vi "Cheak_time.vi"() -> ()   [LabVIEW 2019]
uses:
  <vilib>/Platform/TimedLoop/XDataNode/timing_clust.ctl
  <vilib>/Platform/TimedLoop/XDataNode/nitl_modes.ctl
  <vilib>/Platform/TimedLoop/XDataNode/wakeup.ctl
  <vilib>/FPGAPlugInAG/cRIO-9040/niLvFpga_Open_cRIO-9040.vi
  <vilib>/rvi/interface/common/dynamic/niFpgaDynamicAddResources.vi
  <vilib>/FPGAPlugInAG/Dynamic/niLvFpga_Reset_Dynamic.vi
  <vilib>/FPGAPlugInAG/Dynamic/niLvFpga_Run_Dynamic.vi
  <vilib>/Utility/error.llb/Error Cluster From Error Code.vi
  <vilib>/rvi/errors/niLvFpgaAdjustHostInterfaceError.vi
  <vilib>/FPGAPlugInAG/Dynamic/niLvFpga_Abort_Dynamic.vi
  <vilib>/FPGAPlugInAG/Dynamic/niLvFpga_Close_Dynamic.vi
  <vilib>/rvi/interface/nirviOpenFPGA/nirviOpenFPGA.xnode
  FPGA Bitfiles/hipabvelocitypro_FPGATarget_FPGADATA_ajS4pduxPJ4.lvbitx
  FPGA/FPGA_DATA.vi
  <vilib>/rvi/interface/nirviMethod/nirviMethod.xnode
  <vilib>/Platform/TimedLoop/XDataNode/XDataNode.xnode
  <vilib>/rvi/interface/nirviReadWriteControl/nirviReadWriteControl.xnode
  <vilib>/rvi/interface/nirviCloseFPGA/nirviCloseFPGA.xnode
  <vilib>/Platform/TimedLoop/XDataNode/XDNodeRunTimeDep.lvlib
  NiFpgaLv.dll
  <vilib>/rvi/interface/Simulation/niFpgaSimulationCallBeginRW.vi
panel:
  out "클러스터":T1
  in  "R_velocity":u32
  in  "Temporal parameters_Negative_L":T2={"Onset start"=0.0, "Onset end"=2.0, "Peak start"=10.0, "Release start"=36.0, "slang"=45.0, "Peak end"=34.0}
  in  "L_velocity":u32
  out "Mod1/CAN0":T3={"timestamp high"=0, "timestamp low"=0, "identifier"=0, "type"=enum."Data Frame", "info A"=0, "info B"=0, "data length"=0, "data"=[0, 0, 0, 0, 0, 0, 0, 0]}
  in  "SAVE":bool
  out "웨이브폼 차트 3":T4(graph)
  in  "정지":bool
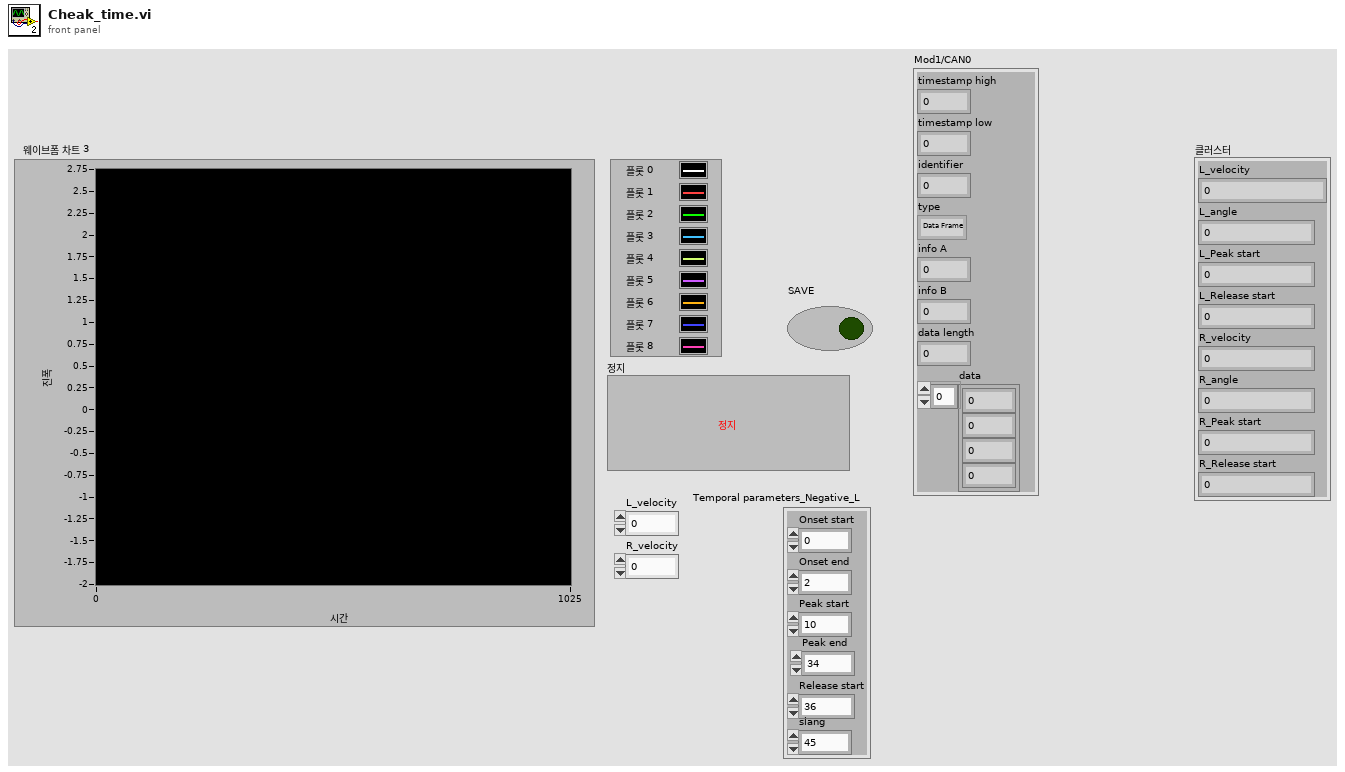
[diagram p1: front panel]
types:
  T1 = cluster{"L_velocity":u32, "L_angle":sgl, "L_Peak start":sgl, "L_Release start":sgl, "R_velocity":u32, "R_angle":sgl, "R_Peak start":sgl, "R_Release start":sgl}
  T2 = cluster{"Onset start":sgl, "Onset end":sgl, "Peak start":sgl, "Release start":sgl, "slang":sgl, "Peak end":sgl}
  T3 = cluster{"timestamp high":u32, "timestamp low":u32, "identifier":u32, "type":enum8{"Data Frame", "Remote Frame", "(reserved)", "(reserved) ", "(reserved)  ", "(reserved)   ", "Bus Error", "Transceiver Fault"}, "info A":u8, "info B":u8, "data length":u8, "data":u8[]}
  T4 = cluster{"[0]":sgl, "[1]":sgl, "[2]":sgl, "[3]":sgl, "[4]":sgl, "[5]":sgl, "[6]":sgl, "[7]":sgl, "[8]":sgl, "[9]":sgl, "[10]":sgl, "[11]":sgl, "[12]":sgl, "[13]":sgl, "[14]":sgl, "[15]":sgl, "[16]":sgl, "[17]":sgl, "[18]":sgl, "[19]":sgl, "[20]":sgl, "[21]":sgl, "[22]":sgl, "[23]":sgl, "[24]":sgl, "[25]":sgl, "[26]":sgl, "[27]":sgl, "[28]":sgl}
  T5 = cluster{"Actual Vel_0":i32, "Actual Pos_0":i32, "Target Pos_0":i32, "Target Vel_0":i32, "Actual Vel_1":i32, "Actual Pos_1":i32, "Target Pos_1":i32, "Target Vel_1":i32, "Target Cur_0":i32, "Target Cur_1":i32, "Q_data":cluster{"Num_L":u32, "Period_L":sgl, "GCP_L":sgl, "Num_R":u32, "Period_R":sgl, "GCP_R":sgl, "FPGA_Data":sgl[], "L_RUN_OK":bool, "R_RUN_OK":bool, "L_ctrl_start":bool, "R_ctrl_start":bool, "Loop time":dbl, "Integrated time":dbl, "Mode":enum16{"Negative", "Positive", "Full"}, "L_acc_mag":sgl, "R_acc_mag":sgl, "L_power_leg":sgl, "R_power_leg":sgl}, "Q_Process":cluster{"LOAD_CELL_PEAK_L":sgl[], "LOAD_CELL_PEAK_R":sgl[], "Flag_L":enum16{"Release_start", "Calculate", "Onset_start", "Peak_start"}, "Flag_R":enum16{"Release_start", "Calculate", "Onset_start", "Peak_start"}, "Status_PS":string, "GCP_1k_R":sgl, "GCP_1k_L":sgl}}[]
  T6 = enum16{"open", "replace", "create", "open or create", "replace or create", "replace or create with confirmation"}
  T7 = typedef "XDNodeRunTimeDep.lvlib/timing_clust.ctl" = cluster{"Expected End [f-1]":u64, "Actual End [f-1]":u64, "Finished Late? [f-1]":bool, "Expected End [i-1]":u64, "Actual End [i-1]":u64, "Finished Late? [i-1]":bool, "Expected Start [i]":u64, "Actual Start [i]":u64, "Expected Start [f]":u64, "Actual Start [f]":u64, "Source Name":string, "Structure Name":string, "Period":i64, "Deadline":i64, "Offset":i64, "Start":i64, "Priority":i32, "Timeout":i32, "Mode":T8, "Wakeup Reason":T9, "Error":errorcluster, "Source Type":string, "Secondary Source Type":string, "Global End Time":u64, "Global Start Time":u64, "Frame Duration":u64, "Iteration Duration":u64, "Assigned CPU":i32, "I/O Scan Engine Mode":u32}
  T8 = typedef "XDNodeRunTimeDep.lvlib/nitl_modes.ctl" = enum32{"No Change", "Process missed periods, maintain original phase", "Discard missed periods, maintain original phase", "Process missed periods, ignore original phase", "Discard missed periods, ignore original phase"}
  T9 = typedef "XDNodeRunTimeDep.lvlib/wakeup.ctl" = enum32{"Normal", "Aborted", "Asynchronous wakeup", "Timing source error", "Timed loop error", "Timeout"}
  T10 = cluster{"timestamp high":u32, "timestamp low":u32, "identifier":u32, "type":enum8{"Data Frame", "Remote Frame", "(reserved)", "(reserved) ", "(reserved)  ", "(reserved)   ", "Bus Error", "Transceiver Fault"}, "info A":u8, "info B":u8, "data length":u8, "data":u8[]}[]
  T11 = cluster{"배열[0]":cluster{"timestamp high":u32, "timestamp low":u32, "identifier":u32, "type":enum8{"Data Frame", "Remote Frame", "(reserved)", "(reserved) ", "(reserved)  ", "(reserved)   ", "Bus Error", "Transceiver Fault"}, "info A":u8, "info B":u8, "data length":u8, "data":u8[]}, "배열[1]":cluster{"timestamp high":u32, "timestamp low":u32, "identifier":u32, "type":enum8{"Data Frame", "Remote Frame", "(reserved)", "(reserved) ", "(reserved)  ", "(reserved)   ", "Bus Error", "Transceiver Fault"}, "info A":u8, "info B":u8, "data length":u8, "data":u8[]}, "배열[2]":cluster{"timestamp high":u32, "timestamp low":u32, "identifier":u32, "type":enum8{"Data Frame", "Remote Frame", "(reserved)", "(reserved) ", "(reserved)  ", "(reserved)   ", "Bus Error", "Transceiver Fault"}, "info A":u8, "info B":u8, "data length":u8, "data":u8[]}, "배열[3]":cluster{"timestamp high":u32, "timestamp low":u32, "identifier":u32, "type":enum8{"Data Frame", "Remote Frame", "(reserved)", "(reserved) ", "(reserved)  ", "(reserved)   ", "Bus Error", "Transceiver Fault"}, "info A":u8, "info B":u8, "data length":u8, "data":u8[]}, "배열[4]":cluster{"timestamp high":u32, "timestamp low":u32, "identifier":u32, "type":enum8{"Data Frame", "Remote Frame", "(reserved)", "(reserved) ", "(reserved)  ", "(reserved)   ", "Bus Error", "Transceiver Fault"}, "info A":u8, "info B":u8, "data length":u8, "data":u8[]}, "배열[5]":cluster{"timestamp high":u32, "timestamp low":u32, "identifier":u32, "type":enum8{"Data Frame", "Remote Frame", "(reserved)", "(reserved) ", "(reserved)  ", "(reserved)   ", "Bus Error", "Transceiver Fault"}, "info A":u8, "info B":u8, "data length":u8, "data":u8[]}, "배열[6]":cluster{"timestamp high":u32, "timestamp low":u32, "identifier":u32, "type":enum8{"Data Frame", "Remote Frame", "(reserved)", "(reserved) ", "(reserved)  ", "(reserved)   ", "Bus Error", "Transceiver Fault"}, "info A":u8, "info B":u8, "data length":u8, "data":u8[]}, "배열[7]":cluster{"timestamp high":u32, "timestamp low":u32, "identifier":u32, "type":enum8{"Data Frame", "Remote Frame", "(reserved)", "(reserved) ", "(reserved)  ", "(reserved)   ", "Bus Error", "Transceiver Fault"}, "info A":u8, "info B":u8, "data length":u8, "data":u8[]}}
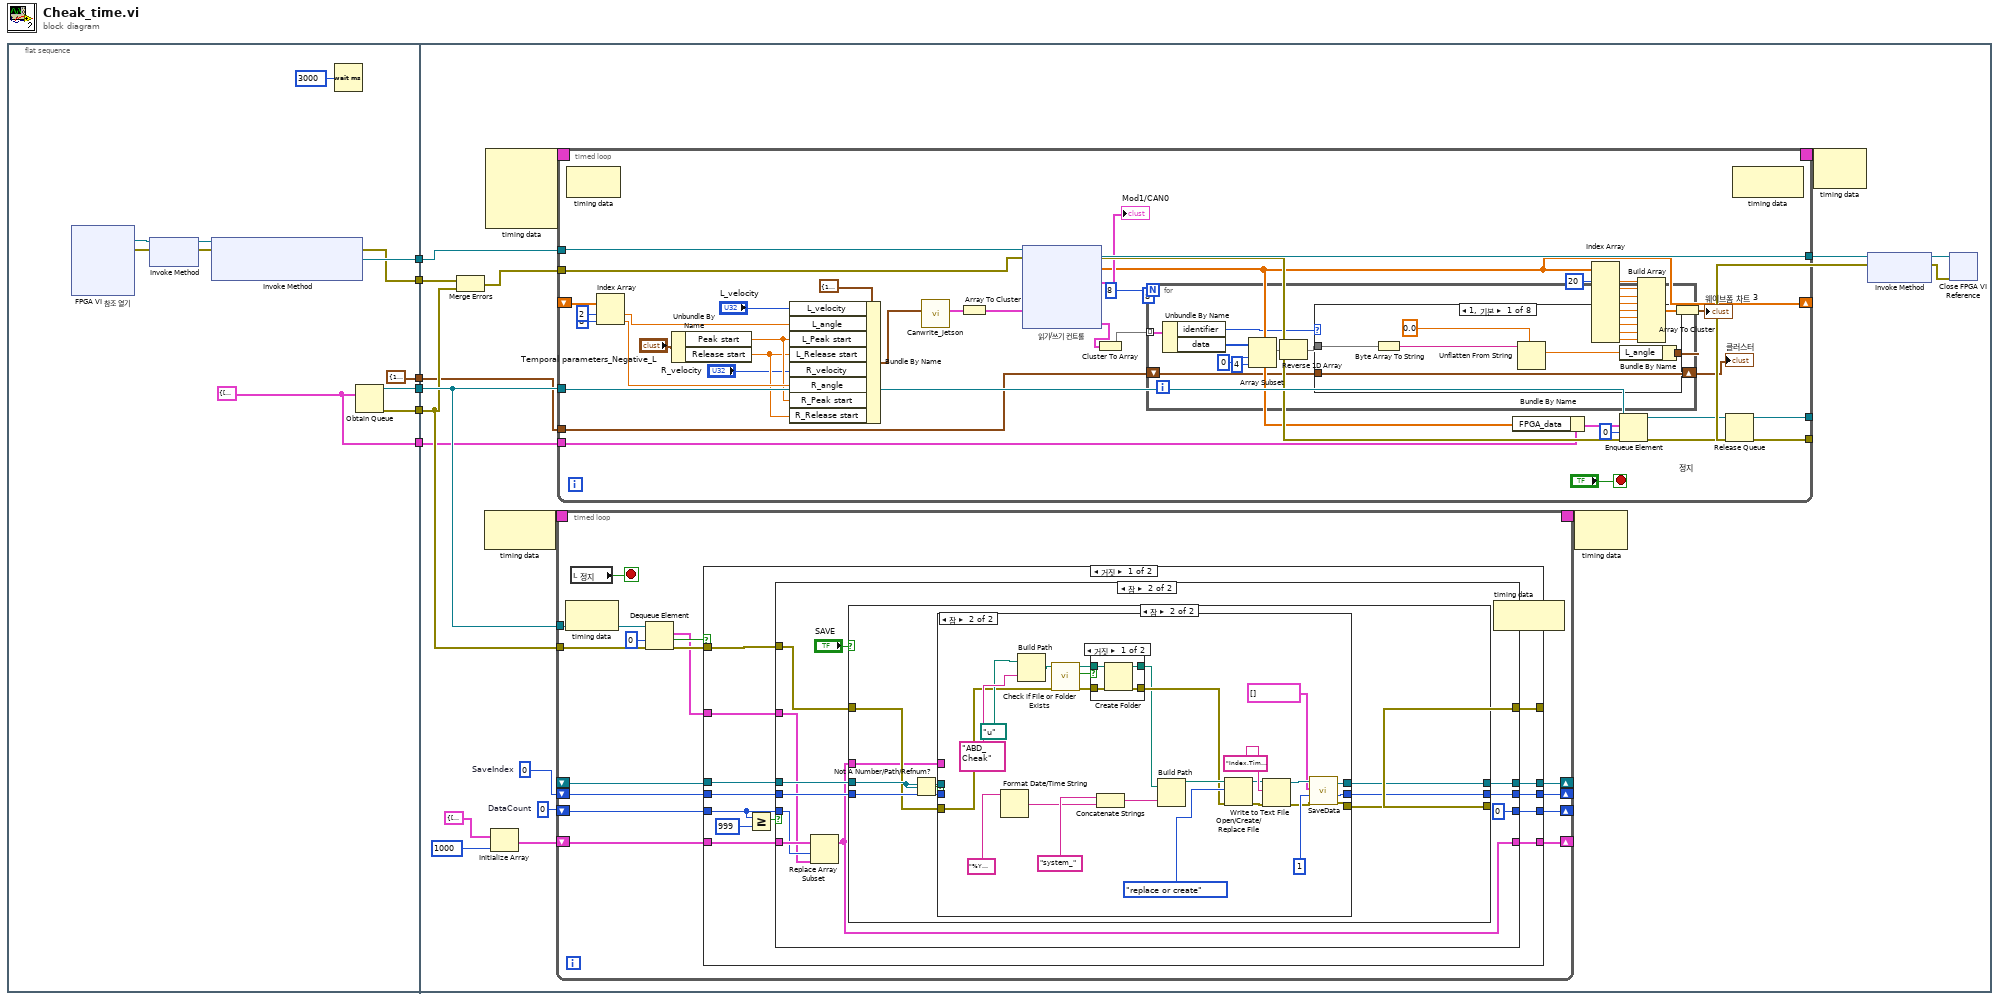
[diagram p0: block diagram]
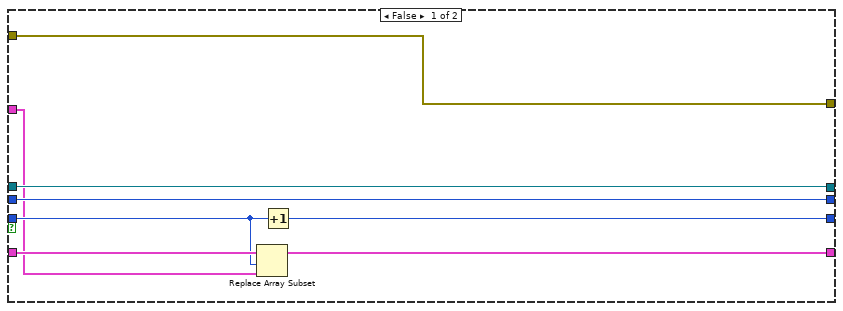
[diagram p2: hidden frame]
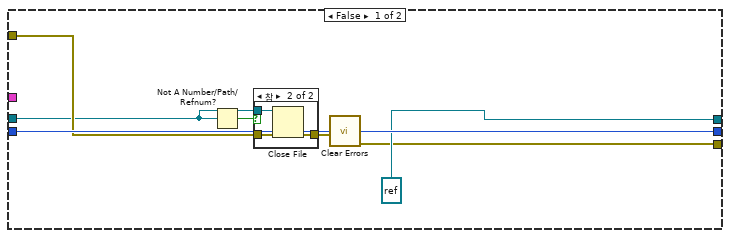
[diagram p3: hidden frame]
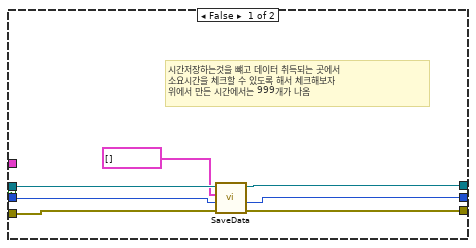
[diagram p5: hidden frame]
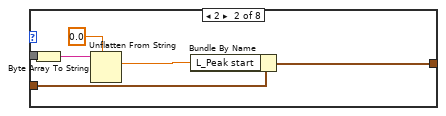
[diagram p8: hidden frame]
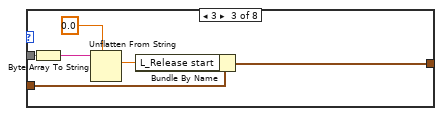
[diagram p9: hidden frame]
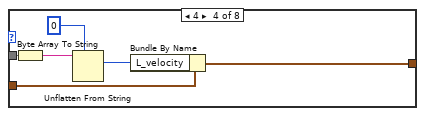
[diagram p10: hidden frame]
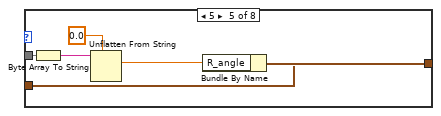
[diagram p11: hidden frame]
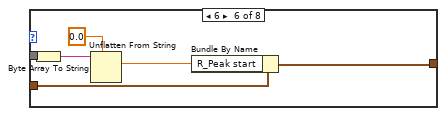
[diagram p12: hidden frame]
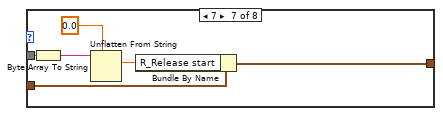
[diagram p13: hidden frame]
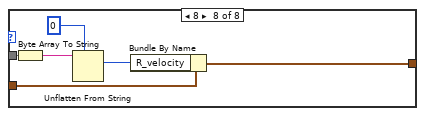
[diagram p14: hidden frame]
diagram:
  n1 = flat-sequence {
    tunnel: [w13] -> w6
    tunnel: [w12] -> w5
    tunnel: [w11] -> w4
    tunnel: [w10] -> w3
    tunnel: [w8] -> w2
    tunnel: [T1 {"L_velocity"=100000, "L_angle"=0.0, "L_Peak start"=10.0, "L_Release start"=36.0, "R_velocity"=100000, "R_angle"=0.0, "R_Peak start"=10.0, "R_Release start"=36.0} ("클러스터")] -> w1
    tunnel: w6 -> [w37]
    tunnel: w5 -> [w30]
    tunnel: w4 -> [w25]
    tunnel: w3 -> [w24]
    tunnel: w2 -> [w22]
    tunnel: w1 -> [w18]
    frame #0 {
      w8 = cluster{"FPGA_data":sgl[]} {"FPGA_data"=[0.0, 0.0, 0.0, 0.0, 0.0, 0.0, 0.0, 0.0, 0.0, 0.0, 0.0, 0.0, 0.0, 0.0, 0.0, 0.0, 0.0, 0.0, 0.0, 0.0, 0.0, 0.0, 0.0, 0.0, 0.0, 0.0, 0.0, 0.0, 0.0]}
      n2 = xnode "FPGA VI 참조 열기"() -> ("FPGA VI 참조 출력"=w17:refnum<k20>, "에러 출력"=w16:errorcluster)  [unwired: 2 in]
      n3 = xnode "Invoke Method"("FPGA VI 참조 입력"=w17, "에러 입력"=w16) -> ("FPGA VI 참조 출력"=w15:refnum<k20>, "에러 출력"=w14:errorcluster)
      n4 = xnode "Invoke Method"("FPGA VI 참조 입력"=w15, "에러 입력"=w14) -> ("FPGA VI 참조 출력"=w13:refnum<k20>, "에러 출력"=w12:errorcluster)  [unwired: 1 in]
      n5 = Wait (ms)(milliseconds to wait=u32 3000 ("대기 시간 (ms)")) -> ()  [unwired: 1 out]
      n6 = Obtain Queue(element data type=w8) -> (queue out=w11:refnum<queue>, error out=w10:errorcluster)  [unwired: 4 in, 1 out]
    }
    frame #1 {
      w19 = 0  # DataCount
      w20 = 0  # SaveIndex
      n7 = Merge Errors(w30, w24) -> (w29:errorcluster)
      n8 = node-c288() -> (w27:T7)  [unwired: 1 in]
      n9 = node-c288() -> (w39:T7)  [unwired: 4 in]
      n10 = Initialize Array(cluster{"FPGA_data":sgl[]} {"FPGA_data"=[0.0, 0.0, 0.0, 0.0, 0.0, 0.0, 0.0, 0.0, 0.0, 0.0, 0.0, 0.0, 0.0, 0.0, 0.0, 0.0, 0.0, 0.0, 0.0, 0.0, 0.0, 0.0, 0.0, 0.0, 0.0, 0.0, 0.0, 0.0, 0.0]}, 1000 ("차원 크기")) -> (w23:cluster{"FPGA_data":sgl[]}[])
      n11 = timed-loop {
        timing: w27 -> [_]
        timing-out: [_] -> w26
        shift-right: [w50] -> _
        shift-left: w20 -> [w53]
        shift-right: [w51] -> _
        shift-left: w19 -> [w54]
        shift-right: [w49] -> _
        shift-left: w23 -> [w52]
        shift-right: [w48] -> _
        shift-left: _ -> [w47]
        tunnel: w25 -> [w45]
        tunnel: w24 -> [w41]
        stop <- w40 stop-if-true
        n12 = node-c288() -> ()  [unwired: 1 in, 1 out]
        n13 = local read "정지"() -> (w40:bool)
        n14 = Dequeue Element(queue=w45, timeout in ms (-1)=0 ("타임아웃(ms) (-1)"), error in (no error)=w41) -> (element=w42:cluster{"FPGA_data":sgl[]}, timed out?=w44:bool, error out=w43:errorcluster)  [unwired: 1 out]
        n15 = case shown="거짓" w44 {
          tunnel: w43 -> [w64 w148]
          tunnel: w54 -> [w62 w146]
          tunnel: w53 -> [w65 w147]
          tunnel: w52 -> [w63 w145]
          tunnel: [w61 w146] -> w51
          tunnel: [w60 w147] -> w50
          tunnel: [w59 w148] -> _
          tunnel: [w58 w145] -> w49
          tunnel: [w57 w149] -> w48
          tunnel: w47 -> [w56 w149]
          tunnel: w42 -> [w55 _]
          frame False {
            n16 = Greater Or Equal?(x=w62, y=999) -> (x >= y?=w66:bool)
            n17 = case shown="참" w66 {
              tunnel: w65 -> [w72 w83]
              tunnel: w64 -> [w71 w81]
              tunnel: w63 -> [w75 w87]
              tunnel: w62 -> [w74 w86]
              tunnel: [w73 0] -> w61
              tunnel: [w72 w82] -> w60
              tunnel: [w71 w78] -> w59
              tunnel: [w70 w77] -> w58
              tunnel: [w69 w80] -> w57
              tunnel: w56 -> [w69 w79]
              tunnel: w55 -> [w68 w76]
              frame False {
                n18 = Replace Array Subset(array=w75, new element=w68, index=w74) -> (w70:cluster{"FPGA_data":sgl[]}[])
                n19 = Increment(x=w74) -> (x+1=w73:i32)
              }
              frame True {
                n20 = Replace Array Subset(array=w87, new element=w76, index=w86) -> (w77:cluster{"FPGA_data":sgl[]}[])
                n21 = case shown="참" "SAVE" {
                  tunnel: w83 -> [w93 w104]
                  tunnel: [w93 w99] -> w82
                  tunnel: w81 -> [w92 w103]
                  tunnel: [refnum<file> refnum ("참조 번호") w101] -> w80
                  tunnel: w79 -> [w90 w105]
                  tunnel: w77 -> [_ w102]
                  tunnel: [w88 w100] -> w78
                  frame False {
                    n22 = Not A Number/Path/Refnum?(number/path/refnum=w90) -> (NaN/Path/Refnum?=w89:bool)
                    n23 = case shown="참" w89 {
                      tunnel: [w95 w98] -> w94
                      tunnel: w92 -> [w95 w97]
                      tunnel: w90 -> [_ w96]
                      frame False {
                      }
                      frame True {
                        n24 = Close File(refnum=w96, error in=w97) -> (error out=w98:errorcluster)  [unwired: 1 out]
                      }
                    }
                    n25 = call <vilib>:"Clear Errors.vi"("error in (no error)"=w94) -> ("error out"=w88:errorcluster)  [unwired: 5 in, 1 out]
                  }
                  frame True {
                    n26 = Not A Number/Path/Refnum?(number/path/refnum=w105) -> (NaN/Path/Refnum?=w106:bool)
                    n27 = case shown="참" w106 {
                      tunnel: w105 -> [w113 _]
                      tunnel: w104 -> [w108 _]
                      tunnel: w103 -> [w109 w128]
                      tunnel: w102 -> [_ _]
                      tunnel: [w112 w119] -> w101
                      tunnel: [w110 w116] -> w100
                      tunnel: [w111 w117] -> w99
                      frame False {
                        # "시간저장하는것을 뺴고 데이터 취득되는 곳에서 \n소요시간을 체크할 수 있도록 해서 체크해보자\n위에서 만든 시간에서는 999개가 나옴"
                        n28 = call "SaveData.vi"("에러 입력"=w109, "Index"=w108, "배열 2"=T5 [], "참조번호"=w113) -> ("에러 출력"=w110:errorcluster, "Index 2"=w111:i32, "참조 번호 출력"=w112:refnum<file>)  [unwired: 5 in]
                      }
                      frame True {
                        n29 = Format Date/Time String(time format string (%c)="%Y%m%d_%H%M%S.csv" ("시간 포맷 문자열 (%c)")) -> (date/time string=w133:string)  [unwired: 2 in]
                        n30 = Build Path(base path=path "u:/" ("베이스 경로"), name or relative path="ABD_Cheak" ("시간 포맷 문자열 (%c)")) -> (appended path=w130:path)
                        n31 = call <vilib>:"Check if File or Folder Exists.vi"("error in (no error)"=w128, "path"=w130) -> ("error out"=w129:errorcluster, "file or folder exists?"=w135:bool, "dup path"=w136:path)  [unwired: 7 in]
                        n32 = case shown="거짓" w135 {
                          tunnel: w136 -> [w142 w144]
                          tunnel: [w141 w144] -> w122
                          tunnel: w129 -> [w140 w143]
                          tunnel: [w139 w143] -> w123
                          frame False {
                            n33 = Create Folder(path (use dialog)=w142, error in=w140) -> (created path=w141:path, error out=w139:errorcluster)  [unwired: 1 in, 1 out]
                          }
                          frame True {
                          }
                        }
                        n34 = Concatenate Strings("system_" ("문자열"), w133) -> (w134:string)
                        n35 = Build Path(base path=w122, name or relative path=w134) -> (appended path=w124:path)
                        n36 = Open/Create/Replace File(file path (use dialog)=w124, error in=w123, operation (0:open)=T6."replace or create" ("동작(0:open)")) -> (refnum out=w121:refnum<file>, error out=w126:errorcluster)  [unwired: 3 in, 1 out]
                        n37 = Write to Text File(file (use dialog)=w121, text="Index,Time,Date,L_Load,R_Load,L_Roll,L_Pitch,L_Yaw,L_accX,L_accY,L_accZ,R_Roll,R_Pitch,R_Yaw,R_accX,R_accY,R_accZ,B_Roll,B_Pitch,B_Yaw,B_accX,B_accY,B_accZ,L_angvel_Rol,L_angvel_Pit,L_angvel_Yaw,R_angvel_Rol,R_angvel_Pit,R_angvel_Yaw,GCP_L,Num_L,Period_L,GCP_R,Num_R,Period_R,Pos_0,Vel_0,T_pos_0,T_vel_0,T_cur_0,Pos_1,Vel_1,T_pos_1,T_vel_1,T_cur_1,GCP_1k_L,GCP_1k_R,L_acc_mag,R_acc_mag,L_run_ok,R_run_ok" ("텍스트"), error in=w126) -> (refnum out=w120:refnum<file>, error out=w115:errorcluster)  [unwired: 1 in, 1 out]
                        n38 = call "SaveData.vi"("에러 입력"=w115, "Index"=1, "배열 2"=T5 [], "참조번호"=w120) -> ("에러 출력"=w116:errorcluster, "Index 2"=w117:i32, "참조 번호 출력"=w119:refnum<file>)  [unwired: 5 in]
                      }
                    }
                  }
                }
              }
            }
          }
          frame True {
          }
        }
        n39 = node-c288() -> ()  [unwired: 1 in, 1 out]
      }
      n40 = timed-loop {
        timing: w39 -> [_]
        timing-out: [_] -> w38
        tunnel: w37 -> [w197]
        tunnel: w29 -> [w196]
        tunnel: [w195] -> w36
        tunnel: [w190] -> w32
        tunnel: w25 -> [w193]
        tunnel: [w192] -> w33
        tunnel: w22 -> [w176]
        shift-right: [w173] -> _
        shift-left: _ -> [w169]
        tunnel: w18 -> [w154]
        stop <- "정지" stop-if-true
        (unwired) 8
        n41 = node-c288() -> ()  [unwired: 1 in, 1 out]
        n42 = Index Array(array=w169, index #1=2 ("인덱스"), index #2=8 ("인덱스")) -> (element #1=w166:sgl, element #2=w165:sgl)
        n43 = Unbundle By Name("Temporal parameters_Negative_L") -> ("Peak start"=w163:sgl, "Release start"=w162:sgl)
        n44 = Bundle By Name(cluster=T1 {"L_velocity"=100000, "L_angle"=0.0, "L_Peak start"=10.0, "L_Release start"=36.0, "R_velocity"=100000, "R_angle"=0.0, "R_Peak start"=10.0, "R_Release start"=36.0} ("클러스터"), "L_velocity"="L_velocity", "L_angle"=w166, "L_Peak start"=w163, "L_Release start"=w162, "R_velocity"="R_velocity", "R_angle"=w165, "R_Peak start"=w163, "R_Release start"=w162) -> (w161:T1)
        n45 = call "Canwrite_jetson.vi"("클러스터"=w161) -> ("배열"=w172:T10)  [unwired: 10 in]
        n46 = Array To Cluster(array=w172) -> (cluster=w159:T11)
        n47 = xnode "읽기/쓰기 컨트롤"("FPGA VI 참조 입력"=w197, "에러 입력"=w196, "Can1 Write"=w159) -> ("FPGA VI 참조 출력"=w195:refnum<k20>, "에러 출력"=w191:errorcluster, "Data"=w173:sgl[], "Mod1/CAN0"=→"Mod1/CAN0":T3, "Can1 Read"=w158:T11)  [unwired: 1 out]
        n48 = Cluster To Array(cluster=w158) -> (array=w157:T10)
        n49 = for {
          N: 8 -> [_]
          tunnel: w157 -> [w206] mode=indexing
          shift-right: [w204] -> w155
          shift-left: w154 -> [w203]
          n50 = Unbundle By Name(w206) -> ("identifier"=w205:u32, "data"=w202:u8[])
          n51 = Array Subset(array=w202, index=0 ("인덱스"), length=4 ("길이")) -> (w199:u8[])
          n52 = Reverse 1D Array(array=w199) -> (reversed array=w198:u8[])
          n53 = case shown="1, 기본" w205 {
            tunnel: w198 -> [w212 w215 w222 w228 w236 w239 w246 w252]
            tunnel: [w208 w214 w221 w227 w232 w238 w245 w251] -> w204
            tunnel: w203 -> [w207 w213 w220 w226 w231 w237 w244 w250]
            frame 1, Default {
              n54 = Byte Array To String(unsigned byte array=w212) -> (string=w211:string)
              n55 = Unflatten From String(type=sgl 0.0, binary string=w211) -> (value=w209:sgl)  [unwired: 3 in, 2 out]
              n56 = Bundle By Name(cluster=w207, "L_angle"=w209) -> (w208:T1)
            }
            frame 2 {
              n57 = Byte Array To String(unsigned byte array=w215) -> (string=w218:string)
              n58 = Unflatten From String(type=sgl 0.0, binary string=w218) -> (value=w216:sgl)  [unwired: 3 in, 2 out]
              n59 = Bundle By Name(cluster=w213, "L_Peak start"=w216) -> (w214:T1)
            }
            frame 3 {
              n60 = Byte Array To String(unsigned byte array=w222) -> (string=w224:string)
              n61 = Unflatten From String(type=sgl 0.0, binary string=w224) -> (value=w223:sgl)  [unwired: 3 in, 2 out]
              n62 = Bundle By Name(cluster=w220, "L_Release start"=w223) -> (w221:T1)
            }
            frame 4 {
              n63 = Byte Array To String(unsigned byte array=w228) -> (string=w230:string)
              n64 = Unflatten From String(type=u32 0, binary string=w230) -> (value=w229:u32)  [unwired: 3 in, 2 out]
              n65 = Bundle By Name(cluster=w226, "L_velocity"=w229) -> (w227:T1)
            }
            frame 5 {
              n66 = Byte Array To String(unsigned byte array=w236) -> (string=w235:string)
              n67 = Unflatten From String(type=sgl 0.0, binary string=w235) -> (value=w233:sgl)  [unwired: 3 in, 2 out]
              n68 = Bundle By Name(cluster=w231, "R_angle"=w233) -> (w232:T1)
            }
            frame 6 {
              n69 = Byte Array To String(unsigned byte array=w239) -> (string=w242:string)
              n70 = Unflatten From String(type=sgl 0.0, binary string=w242) -> (value=w240:sgl)  [unwired: 3 in, 2 out]
              n71 = Bundle By Name(cluster=w237, "R_Peak start"=w240) -> (w238:T1)
            }
            frame 7 {
              n72 = Byte Array To String(unsigned byte array=w246) -> (string=w248:string)
              n73 = Unflatten From String(type=sgl 0.0, binary string=w248) -> (value=w247:sgl)  [unwired: 3 in, 2 out]
              n74 = Bundle By Name(cluster=w244, "R_Release start"=w247) -> (w245:T1)
            }
            frame 8 {
              n75 = Byte Array To String(unsigned byte array=w252) -> (string=w254:string)
              n76 = Unflatten From String(type=u32 0, binary string=w254) -> (value=w253:u32)  [unwired: 3 in, 2 out]
              n77 = Bundle By Name(cluster=w250, "R_velocity"=w253) -> (w251:T1)
            }
          }
        }
        "클러스터" <- w155
        n78 = Bundle By Name(cluster=w176, "FPGA_data"=w173) -> (w175:cluster{"FPGA_data":sgl[]})
        n79 = Index Array(array=w173, index #1=20 ("인덱스")) -> (element #1=w187:sgl, element #2=w186:sgl, element #3=w185:sgl, element #4=w184:sgl, element #5=w183:sgl, element #6=w182:sgl, element #7=w179:sgl, element #8=w178:sgl, element #9=w177:sgl)  [unwired: 8 in]
        n80 = Enqueue Element(queue=w193, element=w175, timeout in ms (-1)=0 ("타임아웃(ms) (-1)"), error in (no error)=w191) -> (queue out=w192:refnum<queue>, error out=w190:errorcluster)  [unwired: 1 out]
        n81 = Build Array(w187, w186, w185, w184, w183, w182, w179, w178, w177) -> (w181:sgl[])
        n82 = Array To Cluster(array=w181) -> (cluster=→"웨이브폼 차트 3":T4)
        n83 = node-c288() -> ()  [unwired: 1 in, 1 out]
      }
      n84 = node-c288(w26) -> ()  [unwired: 1 out]
      n85 = Release Queue(queue=w33, error in (no error)=w32) -> (error out=w31:errorcluster)  [unwired: 1 in, 2 out]
      n86 = node-c288(w38) -> ()  [unwired: 1 out]
      n87 = xnode "Invoke Method"("FPGA VI 참조 입력"=w36, "에러 입력"=w31) -> ("FPGA VI 참조 출력"=w35:refnum<k20>, "에러 출력"=w34:errorcluster)
      n88 = xnode "Close FPGA VI Reference"("FPGA VI 참조 입력"=w35, "에러 입력"=w34) -> ()  [unwired: 1 out]
    }
  }
